vi "Construct_Bad_Track_Without_(111)_Point-1.vi"(6 "[IN] Indexes for Jumps":i32[](array[numeric]), 8 "error IN":errorcluster, 9 "[IN] Index of recon\nstructed tracks":i32, 10 "[IN] Clusters for Re\nconstructed Tracks":T1, 11 "[IN] Still connected\ntracks in group":T2) -> (0 "error OUT":errorcluster, 2 "[OUT] Clusters for Re\nconstructed Tracks":T1)   [LabVIEW 2013]
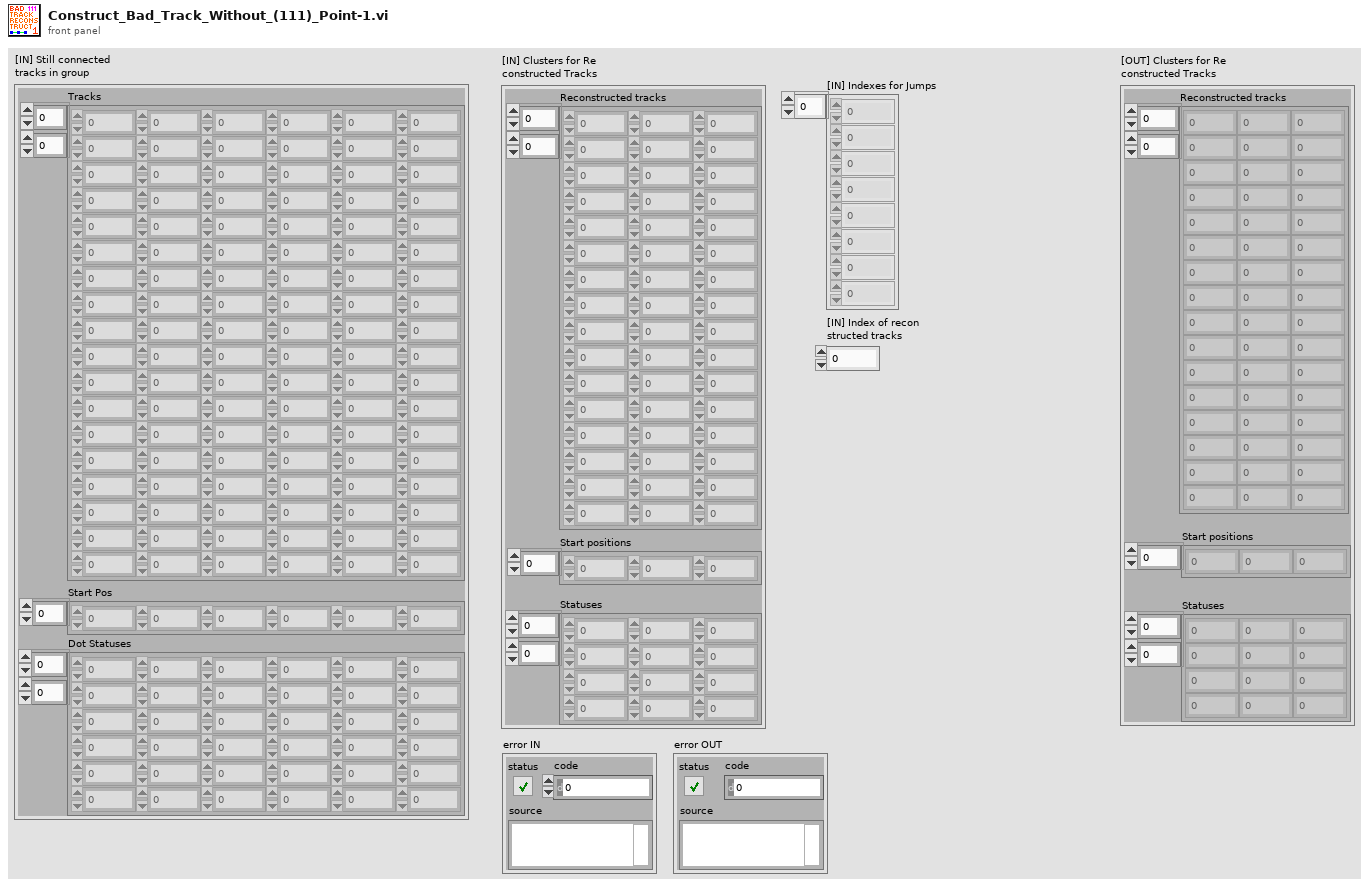
[diagram p1: front panel]
types:
  T1 = cluster{"Reconstructed tracks":dbl[][], "Start positions":i32[], "Statuses":i16[][]}
  T2 = cluster{"Tracks":dbl[][], "Start Pos":i32[], "Dot Statuses":i16[][]}
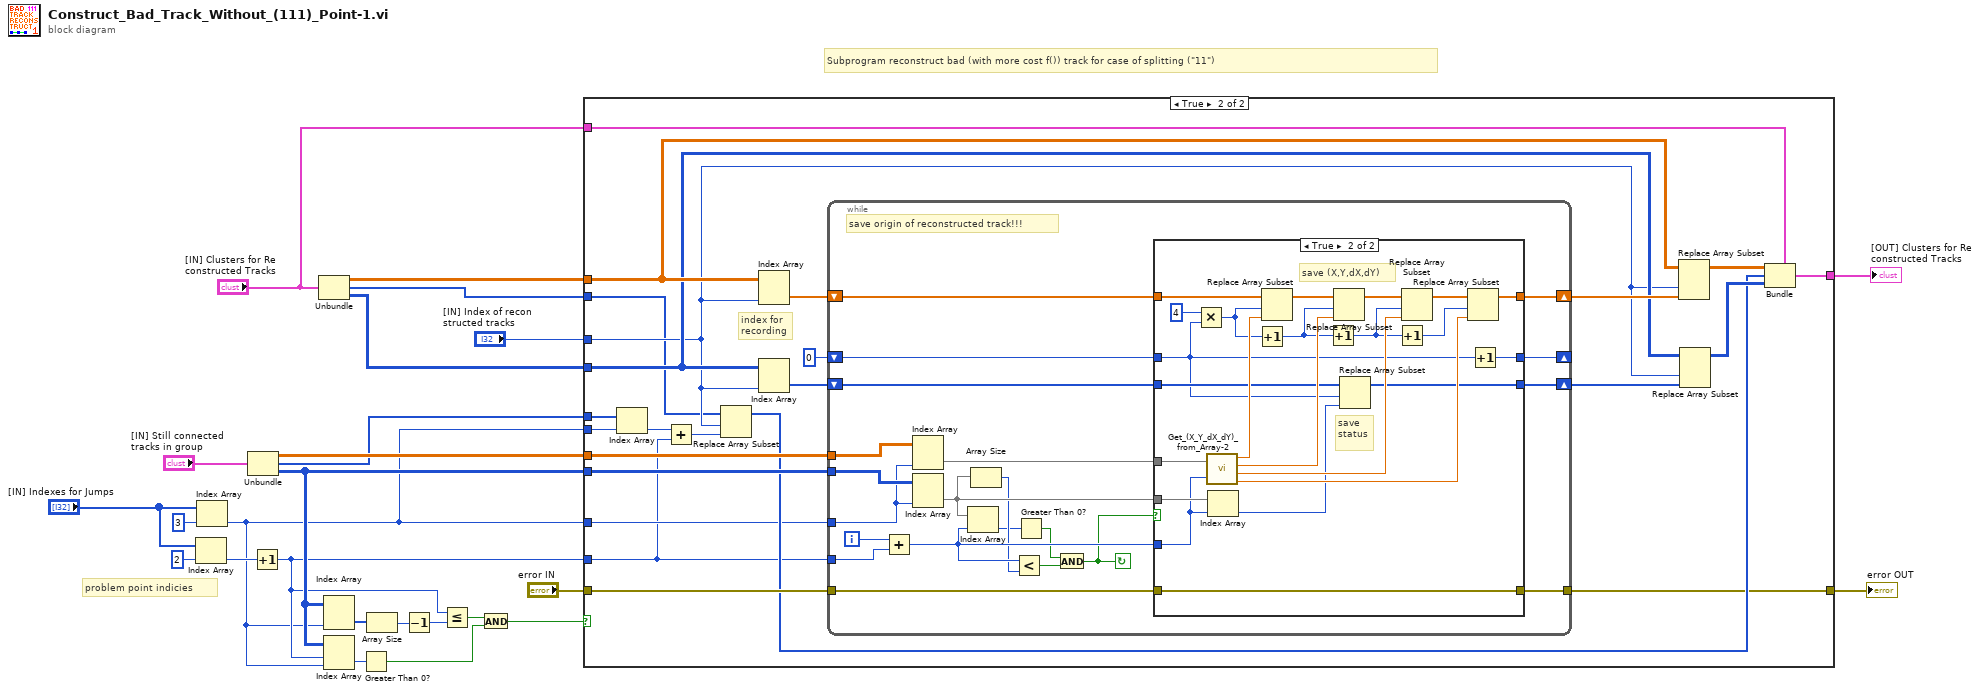
[diagram p0: block diagram]
diagram:
  # "problem point indicies"
  # "Subprogram reconstruct bad (with more cost f()) track for case of splitting (\"11\")"
  n1 = Index Array(array="[IN] Indexes for Jumps", index=2) -> (element=w16:i32)
  n2 = Index Array(array="[IN] Indexes for Jumps", index=3) -> (element=w5:i32)
  n3 = Unbundle("[IN] Still connected\ntracks in group") -> ("Tracks"=w21:dbl[][], "Start Pos"=w2:i32[], "Dot Statuses"=w14:i16[][])
  n4 = Increment(x=w16) -> (x+1=w6:i32)
  n5 = Unbundle("[IN] Clusters for Re\nconstructed Tracks") -> ("Reconstructed tracks"=w20:dbl[][], "Start positions"=w1:i32[], "Statuses"=w19:i16[][])
  n6 = Index Array(array=w14, index (col)=w5) -> (element=w13:i16[])  [unwired: 1 in]
  n7 = Index Array(array=w14, index (row)=w6, index (col)=w5) -> (element=w15:i16)
  n8 = Greater Than 0?(x=w15) -> (x > 0?=w9:bool)
  n9 = Array Size(array=w13) -> (size(s)=w12:i32)
  n10 = Decrement(x=w12) -> (x-1=w11:i32)
  n11 = Less Or Equal?(x=w6, y=w11) -> (x <= y?=w10:bool)
  n12 = And(x=w10, y=w9) -> (x .and. y?=w8:bool)
  n13 = case shown="True" w8 {
    tunnel: w21 -> [_ w48]
    tunnel: w20 -> [_ w41]
    tunnel: w19 -> [_ w40]
    tunnel: "[IN] Index of recon\nstructed tracks" -> [_ w35]
    tunnel: "error IN" -> [w26 w47]
    tunnel: w14 -> [_ w46]
    tunnel: "[IN] Clusters for Re\nconstructed Tracks" -> [w27 w42]
    tunnel: w2 -> [_ w36]
    tunnel: w5 -> [_ w38]
    tunnel: w6 -> [_ w30]
    tunnel: [w27 w32] -> w3
    tunnel: w5 -> [_ w31]
    tunnel: [w26 w29] -> w4
    tunnel: w1 -> [_ w28]
    frame False {
    }
    frame True {
      # "index for\nrecording"
      n14 = Index Array(array=w36, index=w38) -> (element=w37:i32)
      n15 = Add(x=w37, y=w30) -> (x+y=w34:i32)
      n16 = Replace Array Subset(array=w28, new element=w34, index=w35) -> (w33:i32[])
      n17 = Index Array(array=w41, index (col)=w35) -> (element=w51:dbl[])  [unwired: 1 in]
      n18 = Index Array(array=w40, index (col)=w35) -> (element=w50:i16[])  [unwired: 1 in]
      n19 = while {
        tunnel: w30 -> [w59]
        tunnel: w48 -> [w72]
        tunnel: w46 -> [w71]
        tunnel: w31 -> [w70]
        shift-right: [w65] -> w43
        shift-left: w51 -> [w69]
        shift-right: [w63] -> w39
        shift-left: w50 -> [w67]
        shift-right: [w64] -> _
        shift-left: 0 -> [w66]
        tunnel: w47 -> [w62]
        tunnel: [w61] -> w29
        i -> [w60]
        stop <- w52 continue-if-true
        # "save origin of reconstructed track!!!"
        n20 = Add(x=w60, y=w59) -> (x+y=w58:i32)
        n21 = Index Array(array=w72, index (col)=w70) -> (element=w68:dbl[])  [unwired: 1 in]
        n22 = Index Array(array=w71, index (col)=w70) -> (element=w57:i16[])  [unwired: 1 in]
        n23 = Index Array(array=w57, index=w58) -> (element=w54:i16)
        n24 = Array Size(array=w57) -> (size(s)=w56:i32)
        n25 = Less?(x=w58, y=w56) -> (x < y?=w53:bool)
        n26 = Greater Than 0?(x=w54) -> (x > 0?=w55:bool)
        n27 = And(x=w55, y=w53) -> (x .and. y?=w52:bool)
        n28 = case shown="True" w52 {
          tunnel: w69 -> [w76 w97]
          tunnel: w68 -> [_ w99]
          tunnel: w57 -> [_ w98]
          tunnel: w58 -> [_ w82]
          tunnel: w67 -> [w74 w84]
          tunnel: [w74 w81] -> w63
          tunnel: [w76 w80] -> w65
          tunnel: w66 -> [w75 w79]
          tunnel: [w75 w78] -> w64
          tunnel: w62 -> [w73 w77]
          tunnel: [w73 w77] -> w61
          frame False {
          }
          frame True {
            # "save (X,Y,dX,dY)"
            # "save\nstatus"
            n29 = Multiply(x=4, y=w79) -> (x*y=w93:i32)
            n30 = call "Get_(X_Y_dX_dY)_from_Array-2.vi"("(X,Y,dX,dY)"=w99, "Index of Displacement"=w82) -> ("X"=w95:dbl, "Y"=w92:dbl, "dX"=w89:dbl, "dY"=w85:dbl)
            n31 = Index Array(array=w98, index=w82) -> (element=w83:i16)
            n32 = Increment(x=w93) -> (x+1=w90:i32)
            n33 = Replace Array Subset(array=w97, new element=w95, index=w93) -> (w94:dbl[])
            n34 = Increment(x=w90) -> (x+1=w88:i32)
            n35 = Replace Array Subset(array=w94, new element=w92, index=w90) -> (w91:dbl[])
            n36 = Replace Array Subset(array=w84, new element=w83, index=w79) -> (w81:i16[])
            n37 = Increment(x=w88) -> (x+1=w87:i32)
            n38 = Replace Array Subset(array=w91, new element=w89, index=w88) -> (w86:dbl[])
            n39 = Replace Array Subset(array=w86, new element=w85, index=w87) -> (w80:dbl[])
            n40 = Increment(x=w79) -> (x+1=w78:i32)
          }
        }
      }
      n41 = Replace Array Subset(array=w41, new element=w43, index (col)=w35) -> (w44:dbl[][])  [unwired: 1 in]
      n42 = Replace Array Subset(array=w40, new element=w39, index (col)=w35) -> (w45:i16[][])  [unwired: 1 in]
      n43 = Bundle(cluster=w42, "Reconstructed tracks"=w44, "Start positions"=w33, "Statuses"=w45) -> (w32:T1)
    }
  }
  "[OUT] Clusters for Re\nconstructed Tracks" <- w3
  "error OUT" <- w4
